vi "Set Controller Mode and Reference.vi"(8 "error in (no error)":errorcluster, 9 "reference":i32=100, 10 "controller mode":T1=1 items=["Motor Stop", "Positioning-Mode", "Velocity-Mode", "no more action", "set position to reference", "PWM-Mode", "Current-Mode", "Initialize"], 11 "motor slave info in":T2 {"nodeAddr" format="%.0x"}) -> (0 "error out":errorcluster, 2 "valid?":bool, 3 "motor slave info out":T2 {"nodeAddr" format="%.0x"})   [LabVIEW 2017, in "NI_Robotics_KUKA youBot Host.lvlib"]
uses:
  <vilib>/robotics/KUKA youBot/NI_Robotics_KUKA youBot Host.lvlib
  <vilib>/robotics/KUKA youBot/EtherCAT/Motor Slave Info.ctl
  <vilib>/robotics/KUKA youBot/EtherCAT/LowLevel/Mater Handler.ctl
  <vilib>/robotics/KUKA youBot/EtherCAT/Control Mode.ctl
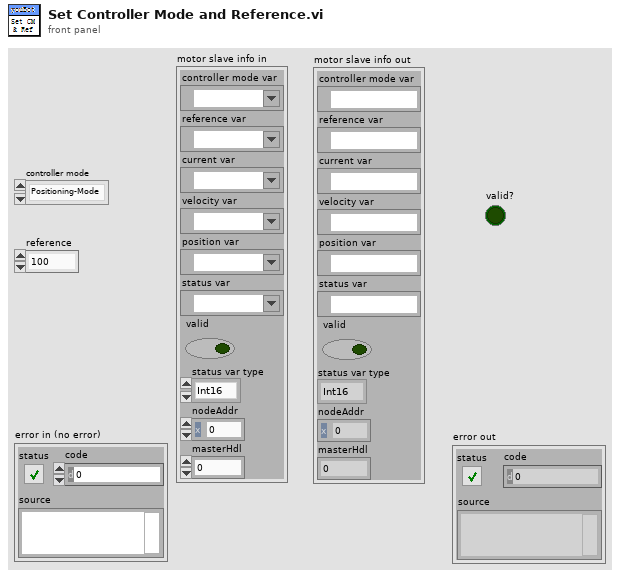
[diagram p1: front panel]
types:
  T1 = typedef "NI_Robotics_KUKA youBot Host.lvlib/Control Mode.ctl" = u8
  T2 = typedef "NI_Robotics_KUKA youBot Host.lvlib/Motor Slave Info.ctl" = cluster{"controller mode var":refnum<k21>, "reference var":refnum<k21>, "current var":refnum<k21>, "velocity var":refnum<k21>, "position var":refnum<k21>, "status var":refnum<k21>, "valid":bool, "status var type":enum16{"Int16", "Int32"}, "nodeAddr":u16, "masterHdl":T3}
  T3 = typedef "NI_Robotics_KUKA youBot Host.lvlib/Mater Handler.ctl" = i32
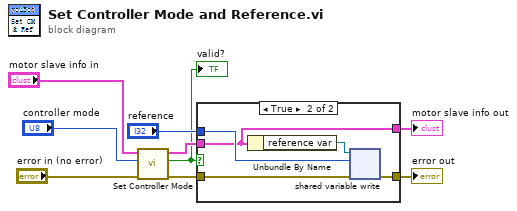
[diagram p0: block diagram]
diagram:
  n1 = call <vilib>:"Set Controller Mode.vi"("error in (no error)"="error in (no error)", "controller mode"="controller mode", "motor slave info in"="motor slave info in") -> ("error out"=w9:errorcluster, "valid?"=w3:bool, "motor slave info out"=w8:T2)  [unwired: 6 in]
  "valid?" <- w3
  n2 = case shown="True" w3 {
    tunnel: "reference" -> [_ w16]
    tunnel: [w11 w15] -> w2
    tunnel: w9 -> [w11 w14]
    tunnel: w8 -> [w10 w13]
    tunnel: [w10 w13] -> w1
    frame False {
    }
    frame True {
      n3 = Unbundle By Name(w13) -> ("reference var"=w12:refnum<k21>)
      n4 = shared-variable-write(w12, w14, w16) -> (w15:errorcluster)  [unwired: 1 out]
    }
  }
  "motor slave info out" <- w1
  "error out" <- w2
